vi "2_6.vi"() -> ()   [LabVIEW 2010]
panel:
  out "x/y":dbl
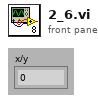
[diagram p1: front panel]
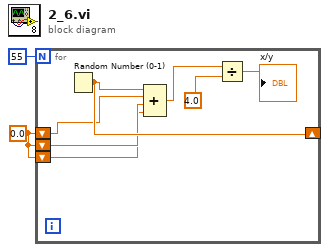
[diagram p0: block diagram]
diagram:
  w1 = 0.0 ("number: 0 to 1")
  n1 = for {
    N: 55 -> [_]
    shift-right: [w6] -> _
    shift-left: w1 -> [w5]
    shift-left: w1 -> [w4]
    shift-left: w1 -> [w3]
    n2 = Random Number (0-1)() -> (number: 0 to 1=w6:dbl)
    n3 = Compound Arithmetic op=ADD(w6, w5, w4, w3) -> (w8:dbl)
    n4 = Divide(x=w8, y=4.0) -> (x/y=→"x/y":dbl)
  }
